vi "test.vi"() -> ()   [LabVIEW 2012]
uses:
  hidapi_32bits.dll
panel:
  out "return type":u32
  in  "timeOfExposure (32 bit)":u32 format="%x"
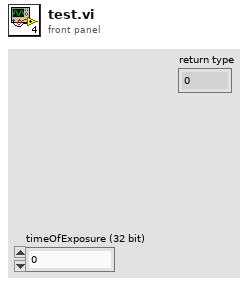
[diagram p1: front panel]
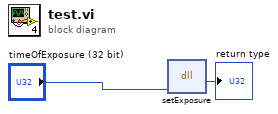
[diagram p0: block diagram]
diagram:
  n1 = dll-call lib="C:/All_Data/mikrocont/Project1/New_controller__Jan_2015/LabView_Aug_2015/hidapi_32bits.dll" fn="setExposure"("timeOfExposure"="timeOfExposure (32 bit)") -> ("return type"=→"return type":u32)  [unwired: 4 in, 2 out]
